vi "Main.vi"(11 "Module Admin":refnum<class "Delacor_lib_QMH_Module Admin.lvclass">) -> ()   [LabVIEW 2024, in "Controller.lvlib"]
doc: "This template is based off of the Queued Message Handler design pattern and the Queued Message Handler project template that ships with LabVIEW.\n\nThe main difference is that the queue is private to this module and communication between modules is performed via Broadcast and Request events.\n\nRequest events are wrapped in public API methods and are handled in the Event Handling Loop (EHL) of this VI. Any module can register for Broadcast events sent by this module. The EHL generates messages based on user interface actions.\n\nThe Message Handling Loop (MHL) processes messages generated by the EHL, or by other messages. The messages are string values, so new messages can be added easily to the Message Cases case structure in the MHL. Each message cluster can also provide an optional value for Message Data, which is a variant that can be converted to whatever message-specific data is required.\n_____\nBased on DQMH Dev Tools: Project Template 7.1.0.1503."
uses:
  Controller.lvlib
  <vilib>/Delacor/Delacor QMH/Libraries/Module Admin_class/Delacor_lib_QMH_Module Admin.lvclass
  Controls/Process state Cluster.ctl
  Controls/Process state enum.ctl
  Module Data--cluster.ctl
  <vilib>/Delacor/Delacor QMH/Libraries/Message Queue_class/Delacor_lib_QMH_Message Queue.lvclass/Delacor_lib_QMH_Message Queue.ctl
  Stop Argument--cluster.ctl
  <vilib>/Delacor/Delacor QMH/Libraries/Module Admin_class/Delacor_lib_QMH_Module Admin.lvclass/Delacor_lib_QMH_Module Admin.ctl
  Login Argument--cluster.ctl
  DB/Controls/Login info.ctl
  DB/Controls/User level.ctl
  Logout Argument--cluster.ctl
  scanner data received Argument--cluster.ctl
  connect all modules Argument--cluster.ctl
  GUI/Controls/Settings.ctl
  <vilib>/Utility/miscctls.llb/LVPointTypeDef.ctl
  <vilib>/Delacor/Delacor QMH/Libraries/Message Queue_class/Delacor_lib_QMH_Enqueue Message (Single).vi
  <vilib>/Delacor/Delacor QMH/Libraries/Module Admin_class/Delacor_lib_QMH_Get External Launch.vi
  <vilib>/Delacor/Delacor QMH/Libraries/Message Queue_class/Delacor_lib_QMH_Message Queue.lvclass
  GUI/GUI.lvlib
  Camera/Camera.lvlib
  DB/DB.lvlib
  Handheld Scanner/Handheld Scanner.lvlib
  PLC/PLC.lvlib
  Aggregation 1/Aggregation 1.lvlib
panel:
  out "scanner read":string
  out "error out":errorcluster
  out "Status":string
  in  "Simulate MHL Error":bool
  in  "Simulate EHL Error":bool
  # "Other processes communicate with this Module via its Public API (wrappers for its Request Events).\n\nThis Module communicates with other processes via its Broadcast Events.\nAny process that wants to receive these messages can register for this module's Broadcast events."
  # "This template is for the DQMH framework. See the block diagram for more information on how to use this template."
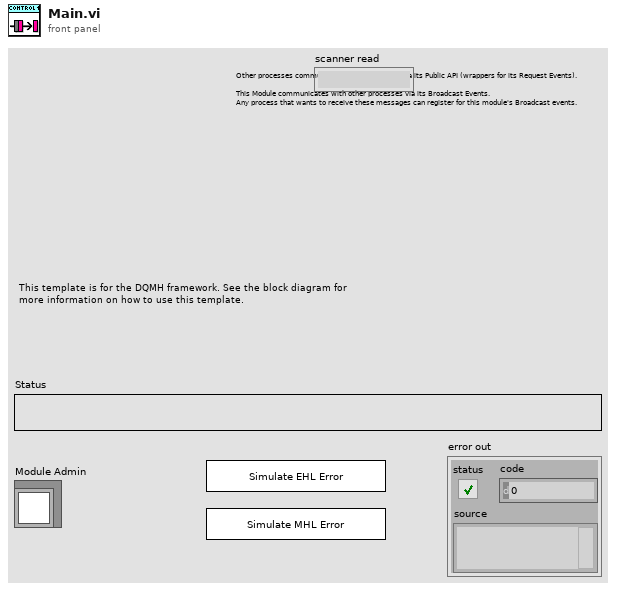
[diagram p1: front panel]
types:
  T1 = typedef "Process state Cluster.ctl" = cluster{T2, variant}
  T2 = typedef "Process state enum.ctl" = enum16{"init", "login", "Agg start", "Agg stop", "logout", "Terminate"}
  T3 = typedef "Controller.lvlib/Request Events--cluster.ctl" = cluster{"Stop Module":refnum<user-event>, "Show Panel":refnum<user-event>, "Hide Panel":refnum<user-event>, "Get Module Execution Status":refnum<user-event>, "Show Diagram":refnum<user-event>, "Login":refnum<user-event>, "Logout":refnum<user-event>, "scanner data received":refnum<user-event>, "connect all modules":refnum<user-event>}
  T4 = typedef "Controller.lvlib/Module Data--cluster.ctl" = cluster{"Status":string}
  T5 = enum32{"invalid lock state", "Not Locked", "Locked (No Password)", "Password-protected"}
  T6 = typedef "Controller.lvlib/Stop Argument--cluster.ctl" = cluster{"Origin":string, "Exit via Stop Module Req?":bool, "Wait for Module to stop?":bool}
  T7 = typedef "Controller.lvlib/Login Argument--cluster.ctl" = cluster{"Login info":T8}
  T8 = typedef "Login info.ctl" = cluster{"User Name":string, "User level":T9}
  T9 = typedef "User level.ctl" = enum16{"Operator", "Admin"}
  T10 = typedef "Controller.lvlib/Logout Argument--cluster.ctl" = cluster{"Boolean":bool}
  T11 = typedef "Controller.lvlib/scanner data received Argument--cluster.ctl" = cluster{"scanner read":string}
  T12 = typedef "Controller.lvlib/connect all modules Argument--cluster.ctl" = cluster{"Settings":T13}
  T13 = typedef "Settings.ctl" = cluster{"Camera 1 IP":string, "Camera 2 IP":string, "Printer 1 IP":string, "Printer 2 IP":string, "Level 2 Scanner COM":refnum<visa-resource-name>, "PLC Port":dbl, "PLC IP":string, "Handheld Scanner COM":refnum<visa-resource-name>, "Printer2 Port":dbl, "Cam1 send port ":dbl, "Cam1 recv port":dbl, "Cam2 send port":dbl, "Cam recv port":dbl, "Printer1 Port":dbl}
  T14 = typedef "LVPointTypeDef.ctl" = cluster{"Horizontal":i16, "Vertical":i16}
  T15 = enum32{"Invalid", "Standard", "Closed", "Hidden", "Minimized", "Maximized"}
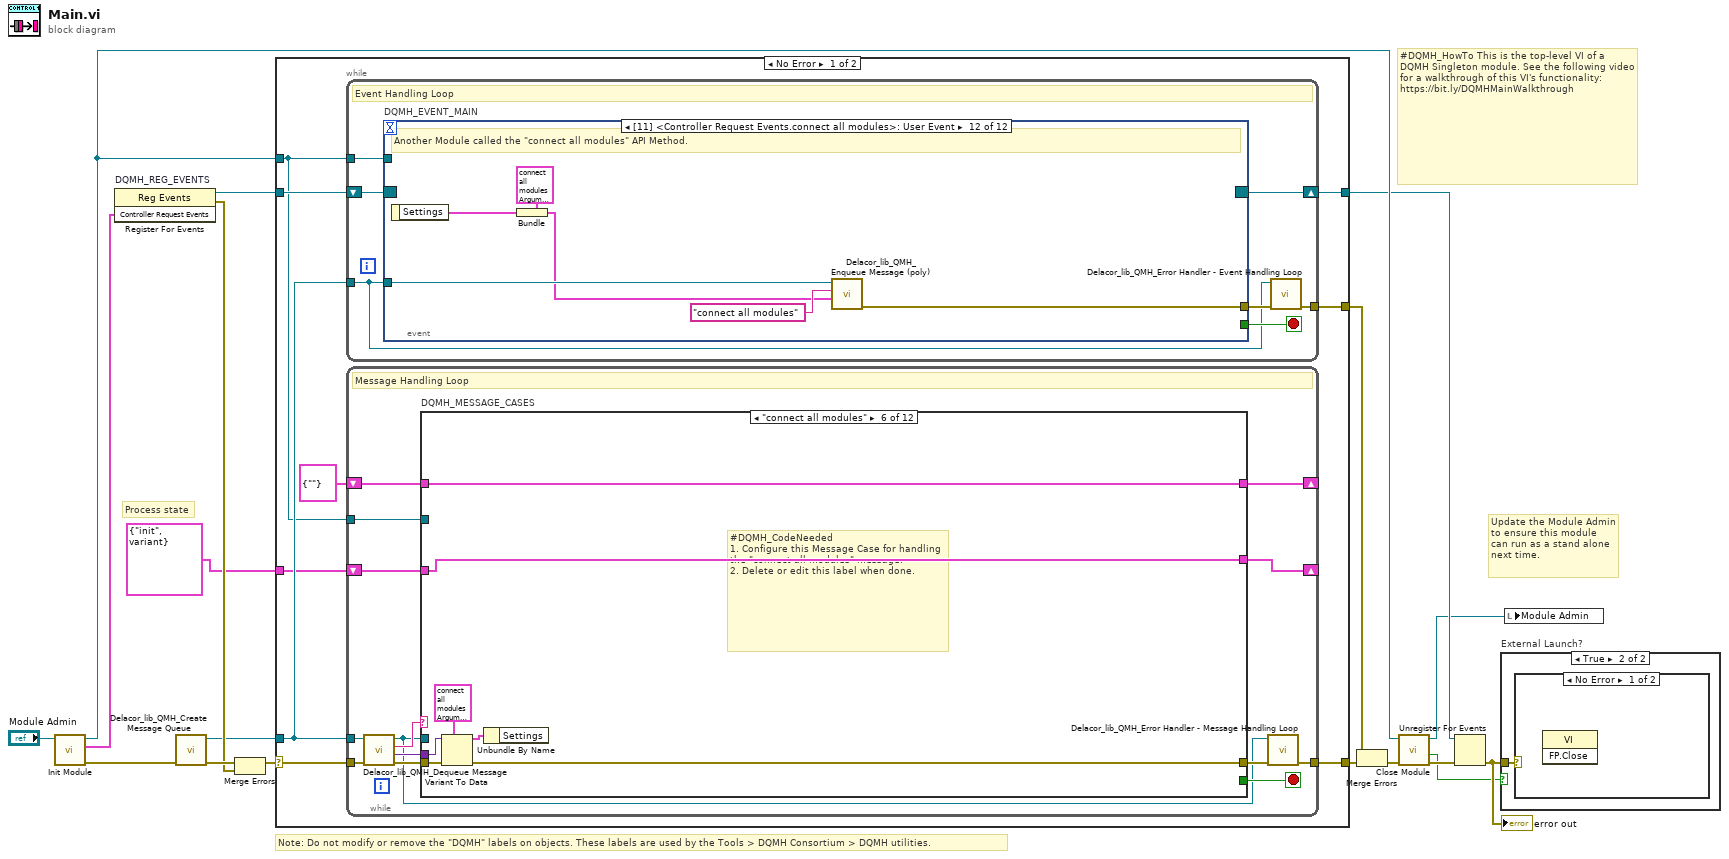
[diagram p0: block diagram]
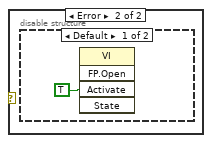
[diagram p3: hidden frame]
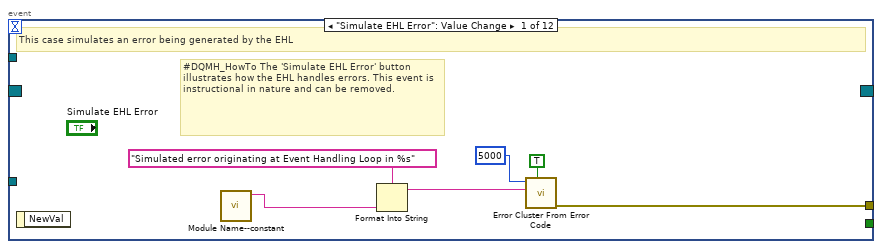
[diagram p5: hidden frame]
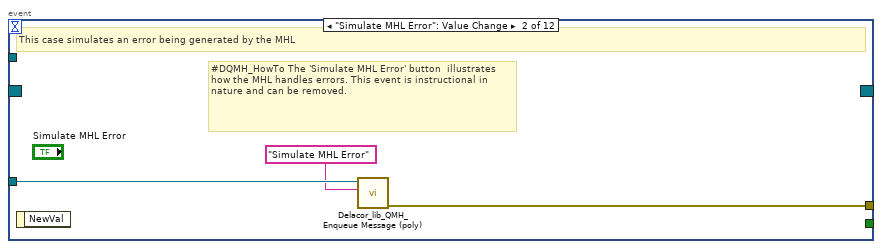
[diagram p6: hidden frame]
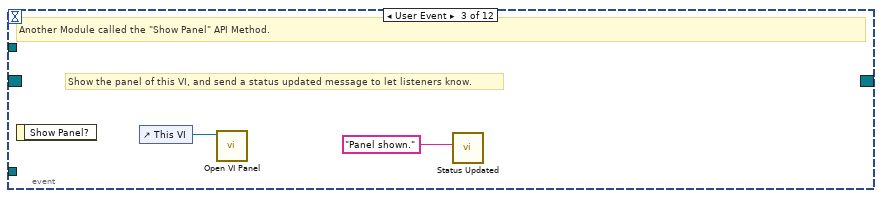
[diagram p7: hidden frame]
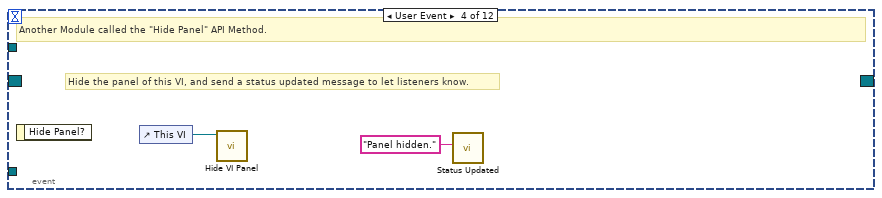
[diagram p8: hidden frame]
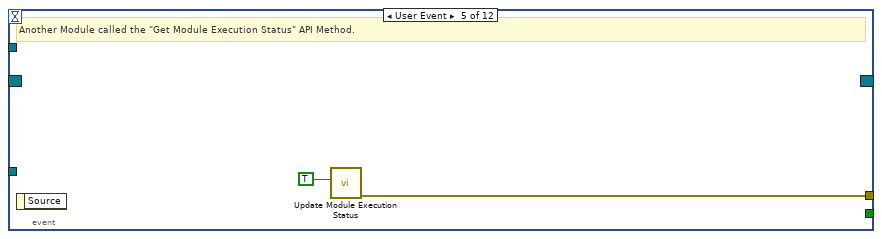
[diagram p9: hidden frame]
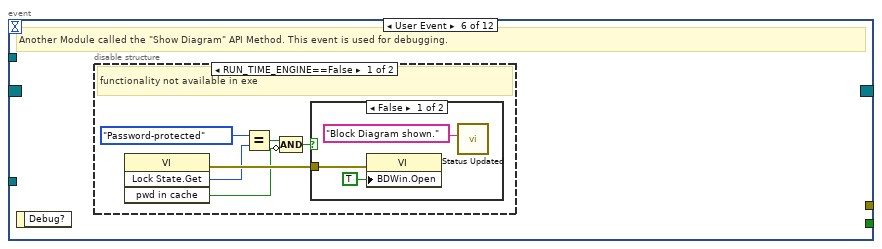
[diagram p10: hidden frame]
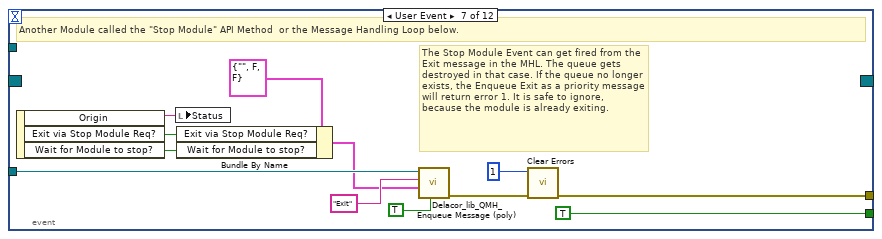
[diagram p13: hidden frame]
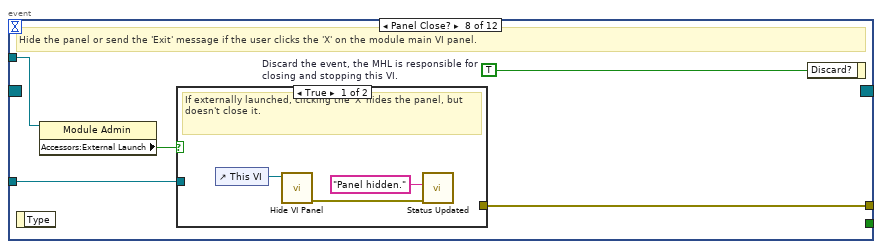
[diagram p14: hidden frame]
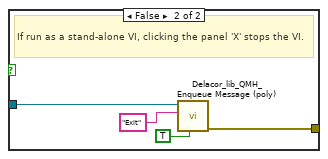
[diagram p15: hidden frame]
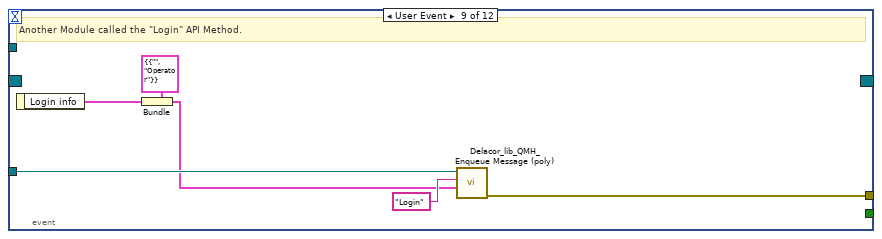
[diagram p16: hidden frame]
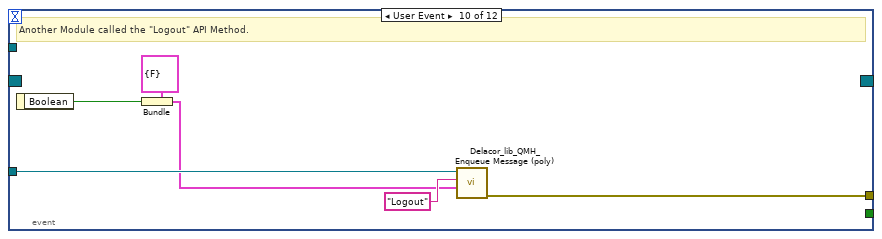
[diagram p17: hidden frame]
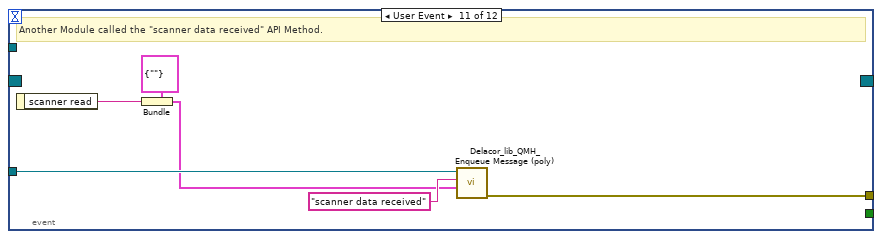
[diagram p18: hidden frame]
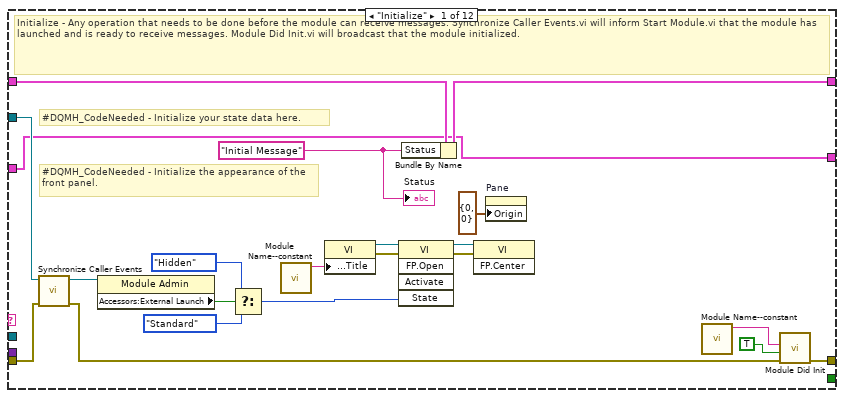
[diagram p19: hidden frame]
diagram:
  # "Process state"
  # "#DQMH_HowTo This is the top-level VI of a DQMH Singleton module. See the following video for a walkthrough of this VI's functionality: https://bit.ly/DQMHMainWalkthrough"
  # "Note: Do not modify or remove the \"DQMH\" labels on objects. These labels are used by the Tools > DQMH Consortium > DQMH utilities."
  # "Update the Module Admin to ensure this module can run as a stand alone next time."
  n1 = call "Init Module.vi"("Singleton Module Admin in"="Module Admin") -> ("error out"=w17:errorcluster, "Controller Request Events"=w6:T3, "Singleton Module Admin out"=w9:refnum<class "Delacor_lib_QMH_Module Admin.lvclass">)  [unwired: 8 in]
  n2 = register-events "DQMH_REG_EVENTS"(w6) -> (reference out=w7:refnum<event-registration>, error out=w10:errorcluster)  [unwired: 2 in]
  n3 = call <vilib>:"Delacor_lib_QMH_Create Message Queue.vi"("error in"=w17) -> ("error out"=w12:errorcluster, "Message Queue"=w5:refnum<class "Delacor_lib_QMH_Message Queue.lvclass">)  [unwired: 9 in]
  n4 = Merge Errors(w12, w10) -> (w11:errorcluster)
  n5 = case shown="No Error" w11 {
    selector: w11 -> [w25 w245]
    tunnel: [w27 w244] -> w18
    tunnel: [w24 w243] -> w8
    tunnel: w7 -> [w22 w243]
    tunnel: w5 -> [w21 w238]
    tunnel: [w26 _] -> w15
    tunnel: w9 -> [w20 w239]
    tunnel: T1 {enum."init", variant} -> [w19 _]
    frame No Error {
      n6 = while {
        tunnel: w21 -> [w28]
        shift-right: [w31] -> w24
        shift-left: w22 -> [w32]
        tunnel: [w33] -> w26
        tunnel: w20 -> [w29]
        stop <- w30 stop-if-true
        # "Event Handling Loop"
        n7 = event "DQMH_EVENT_MAIN" shown="[11] <Controller Request Events.connect all modules>: User Event" {
          selector: w32 -> [_ _ _ _ _ _ _ _ _ _ _ _]
          dyn-events: [_ _ _ _ _ _ _ _ _ _ _ _] -> w31
          timeout: _ -> [_ _ _ _ _ _ _ _ _ _ _ _]
          tunnel: [_ _ _ _ _ _ TRUE ("Discard?") _ _ _ _ _] -> w30
          tunnel: w28 -> [_ w42 _ _ _ _ w66 w73 w88 w94 w100 w106]
          tunnel: [w40 w43 _ _ w49 _ w69 w75 w83 w89 w95 w101] -> w34
          tunnel: w29 -> [_ _ _ _ _ _ _ w72 _ _ _ _]
          event "Simulate EHL Error": Value Change {
            # "#DQMH_HowTo The 'Simulate EHL Error' button  illustrates how the EHL handles errors. This event is instructional in nature and can be removed."
            # "This case simulates an error being generated by the EHL"
            n8 = event-data() -> ()  [unwired: 1 in, 1 out]
            n9 = call "Module Name--constant.vi"() -> ("Module Name"=w37:string)  [unwired: 11 in]
            n10 = Format Into String(format string="Simulated error originating at Event Handling Loop in %s", w37) -> (resulting string=w38:string)  [unwired: 2 in, 1 out]
            n11 = call <vilib>:"Error Cluster From Error Code.vi"("show call chain? (False)"=TRUE, "error message (\"\")"=w38, "error code (0)"=5000) -> ("error out"=w40:errorcluster)  [unwired: 6 in]
          }
          event "Simulate MHL Error": Value Change {
            # "#DQMH_HowTo The 'Simulate MHL Error' button  illustrates how the MHL handles errors. This event is instructional in nature and can be removed."
            # "This case simulates an error being generated by the MHL"
            n12 = event-data() -> ()  [unwired: 1 in, 1 out]
            n13 = call-poly <vilib>:"Delacor_lib_QMH_Enqueue Message (poly).vi"("Message"="Simulate MHL Error", "Message Queue in"=w42) -> ("error out"=w43:errorcluster)  [unwired: 8 in, 1 out]
          }
          event User Event {
            # "Show the panel of this VI, and send a status updated message to let listeners know."
            # "Another Module called the \"Show Panel\" API Method."
            n14 = event-data() -> ()  [unwired: 1 in, 1 out]
            n15 = control-ref of="This VI"() -> (w45:refnum<vi>)
            n16 = call "Open VI Panel.vi"("VI"=w45) -> ()  [unwired: 10 in, 1 out]
            n17 = call "Status Updated.vi"("Status"="Panel shown." ("format string")) -> ()  [unwired: 10 in, 1 out]
          }
          event User Event {
            # "Hide the panel of this VI, and send a status updated message to let listeners know."
            # "Another Module called the \"Hide Panel\" API Method."
            n18 = event-data() -> ()  [unwired: 1 in, 1 out]
            n19 = control-ref of="This VI"() -> (w47:refnum<vi>)
            n20 = call "Hide VI Panel.vi"("VI"=w47) -> ()  [unwired: 10 in, 1 out]
            n21 = call "Status Updated.vi"("Status"="Panel hidden." ("format string")) -> ()  [unwired: 10 in, 1 out]
          }
          event User Event {
            # "Another Module called the \"Get Module Execution Status\" API Method."
            n22 = event-data() -> ()  [unwired: 1 in, 1 out]
            n23 = call "Update Module Execution Status.vi"("Running?"=TRUE) -> ("error out"=w49:errorcluster)  [unwired: 10 in]
          }
          event User Event {
            # "Another Module called the \"Show Diagram\" API Method. This event is used for debugging."
            n24 = event-data() -> ()  [unwired: 1 in, 1 out]
            n25 = disable-structure shown="RUN_TIME_ENGINE==False" {
              frame condition #0 (active) {
                # "functionality not available in exe"
                n26 = invoke on="Invoke Node" class="VI" method="Lock State.Get"() -> (error out=w55:errorcluster, "Get Lock State"=w54:T5, "pwd in cache"=w51:bool)  [unwired: 4 in, 1 out]
                n27 = Equal?(x=T5."Password-protected", y=w54) -> (x = y?=w52:bool)
                n28 = Compound Arithmetic op=AND(w52, invert w51) -> (w50:bool)
                n29 = case shown="False" w50 {
                  tunnel: w55 -> [w58 _]
                  frame False {
                    n30 = property on="Property Node" class="VI"(error in=w58, "BDWin.Open"=TRUE ("Block Diagram Window:Open")) -> ()  [unwired: 1 in, 2 out]
                    n31 = call "Status Updated.vi"("Status"="Block Diagram shown." ("format string")) -> ()  [unwired: 10 in, 1 out]
                  }
                  frame True {
                    # "Password-protected VI, and the password is not in the cache. Do not show the diagram."
                  }
                }
              }
              frame condition #1 {
              }
            }
          }
          event User Event {
            # "The Stop Module Event can get fired from the Exit message in the MHL. The queue gets destroyed in that case. If the queue no longer exists, the Enqueue Exit as a priority message will return error 1. It is safe to ignore, because the module is already exiting."
            # "Another Module called the \"Stop Module\" API Method  or the Message Handling Loop below."
            n32 = event-data() -> ("Origin"=w65:string, "Exit via Stop Module Req?"=w61:bool, "Wait for Module to stop?"=w60:bool)  [unwired: 1 in]
            n33 = local write "Status"(w65) -> ()
            n34 = Bundle By Name(cluster=T6 {"Origin"="", "Exit via Stop Module Req?"=FALSE, "Wait for Module to stop?"=FALSE} ("Stop Argument"), "Exit via Stop Module Req?"=w61, "Wait for Module to stop?"=w60) -> (w59:T6)
            n35 = call-poly <vilib>:"Delacor_lib_QMH_Enqueue Message (poly).vi"("Priority Message? (F)"=TRUE, "Message Data"=w59, "Message"="Exit", "Message Queue in"=w66) -> ("error out"=w70:errorcluster)  [unwired: 6 in, 1 out]
            n36 = call <vilib>:"Clear Errors.vi"("error in (no error)"=w70, "specific error code to clear (0: all)"=1) -> ("error out"=w69:errorcluster)  [unwired: 4 in, 1 out]
          }
          event Panel Close? {
            w74 = TRUE  # Discard the event, the MHL is responsible for closing and stopping this VI.
            # "Hide the panel or send the 'Exit' message if the user clicks the 'X' on the module main VI panel."
            n37 = event-data() -> ()  [unwired: 1 in, 1 out]
            n38 = property on="Property Node" class="Module Admin"(reference=w72) -> ("Accessors:External Launch"=w71:bool)  [unwired: 1 in, 2 out]
            n39 = case shown="True" w71 {
              tunnel: w73 -> [_ w81]
              tunnel: [_ w82] -> w75
              frame True {
                # "If externally launched, clicking the 'X' hides the panel, but doesn't close it."
                n40 = control-ref of="This VI"() -> (w78:refnum<vi>)
                n41 = call "Hide VI Panel.vi"("VI"=w78) -> ("error out"=w76:errorcluster)  [unwired: 10 in]
                n42 = call "Status Updated.vi"("error in"=w76, "Status"="Panel hidden." ("format string")) -> ()  [unwired: 9 in, 1 out]
              }
              frame False {
                # "If run as a stand-alone VI, clicking the panel 'X' stops the VI."
                n43 = call-poly <vilib>:"Delacor_lib_QMH_Enqueue Message (poly).vi"("Priority Message? (F)"=TRUE, "Message"="Exit", "Message Queue in"=w81) -> ("error out"=w82:errorcluster)  [unwired: 7 in, 1 out]
              }
            }
            n44 = event-data ("Event Filter Node")("Discard?"=w74) -> ()  [unwired: 1 in, 1 out]
          }
          event User Event {
            # "Another Module called the \"Login\" API Method."
            n45 = event-data() -> ("Login info"=w84:T8)  [unwired: 1 in]
            n46 = Bundle(cluster=T7 {"Login info"={"User Name"="", "User level"=enum."Operator"}} ("Login Argument"), "Login info"=w84) -> (w85:T7)
            n47 = call-poly <vilib>:"Delacor_lib_QMH_Enqueue Message (poly).vi"("Message Data"=w85, "Message"="Login", "Message Queue in"=w88) -> ("error out"=w83:errorcluster)  [unwired: 7 in, 1 out]
          }
          event User Event {
            # "Another Module called the \"Logout\" API Method."
            n48 = event-data() -> ("Boolean"=w90:bool)  [unwired: 1 in]
            n49 = Bundle(cluster=T10 {"Boolean"=FALSE} ("Logout Argument"), "Boolean"=w90) -> (w91:T10)
            n50 = call-poly <vilib>:"Delacor_lib_QMH_Enqueue Message (poly).vi"("Message Data"=w91, "Message"="Logout", "Message Queue in"=w94) -> ("error out"=w89:errorcluster)  [unwired: 7 in, 1 out]
          }
          event User Event {
            # "Another Module called the \"scanner data received\" API Method."
            n51 = event-data() -> ("scanner read"=w96:string)  [unwired: 1 in]
            n52 = Bundle(cluster=T11 {"scanner read"=""} ("scanner data received Argument"), "scanner read"=w96) -> (w97:T11)
            n53 = call-poly <vilib>:"Delacor_lib_QMH_Enqueue Message (poly).vi"("Message Data"=w97, "Message"="scanner data received", "Message Queue in"=w100) -> ("error out"=w95:errorcluster)  [unwired: 7 in, 1 out]
          }
          event User Event {
            # "Another Module called the \"connect all modules\" API Method."
            n54 = event-data() -> ("Settings"=w102:T13)  [unwired: 1 in]
            n55 = Bundle(cluster=T12 {"Settings"={"Camera 1 IP"="", "Camera 2 IP"="", "Printer 1 IP"="", "Printer 2 IP"="", "Level 2 Scanner COM"="", "PLC Port"=0.0, "PLC IP"="", "Handheld Scanner COM"="", "Printer2 Port"=0.0, "Cam1 send port "=0.0, "Cam1 recv port"=0.0, "Cam2 send port"=0.0, "Cam recv port"=0.0, "Printer1 Port"=0.0}} ("connect all modules Argument"), "Settings"=w102) -> (w103:T12)
            n56 = call-poly <vilib>:"Delacor_lib_QMH_Enqueue Message (poly).vi"("Message Data"=w103, "Message"="connect all modules", "Message Queue in"=w106) -> ("error out"=w101:errorcluster)  [unwired: 7 in, 1 out]
          }
        }
        n57 = call-dynamic "Delacor_lib_QMH_Error Handler - Event Handling Loop.vi"("error in"=w34, "Message Queue in"=w28) -> ("dup error in"=w33:errorcluster)  [unwired: 8 in, 1 out]
      }
      n58 = while {
        tunnel: w21 -> [w109]
        shift-right: [w117] -> _
        shift-left: T4 {"Status"=""} ("Data Cluster") -> [w118]
        tunnel: w25 -> [w120]
        tunnel: [w112] -> w27
        tunnel: w20 -> [w113]
        shift-right: [w107] -> _
        shift-left: w19 -> [w108]
        stop <- w116 stop-if-true
        # "Message Handling Loop"
        n59 = call-dynamic "Delacor_lib_QMH_Dequeue Message.vi"("error in"=w120, "Message Queue in"=w109) -> ("error out"=w119:errorcluster, "Message Data"=w114:variant, "Message"=w115:string, "Message Queue out"=w110:refnum<class "Delacor_lib_QMH_Message Queue.lvclass">)  [unwired: 6 in]
        n60 = case "DQMH_MESSAGE_CASES" shown="\"connect all modules\"" w115 {
          selector: w115 -> [_ _ _ _ _ _ _ _ _ _ _ w233]
          tunnel: w110 -> [_ _ _ _ _ _ _ _ _ w196 w220 _]
          tunnel: w119 -> [w139 w144 w152 w159 w167 w174 w178 w181 w191 w203 w226 w236]
          tunnel: [w137 w144 w150 w157 w165 w171 w177 w181 w190 w199 w221 w237] -> w111
          tunnel: w118 -> [w128 w143 w151 w158 w166 w173 w176 w180 w188 w198 w219 w234]
          tunnel: [w127 w143 w151 w158 w166 w173 w176 w180 w188 w198 w219 w234] -> w117
          tunnel: [_ _ _ _ _ _ _ _ _ _ w218 _] -> w116
          tunnel: w114 -> [_ _ w149 w156 w164 w170 _ _ _ w197 w217 _]
          tunnel: w113 -> [w129 _ _ _ _ _ _ _ _ w195 w212 _]
          tunnel: w108 -> [w121 w142 _ w153 w160 w172 w175 w179 w182 w192 w210 w227]
          tunnel: [w121 w142 T1 {enum."login", variant} w153 w160 w172 w175 w179 w182 w192 w210 w227] -> w107
          frame "Initialize" {
            w123 = "Initial Message" ("Initial Message")
            # "#DQMH_CodeNeeded - Initialize the appearance of the front panel."
            # "#DQMH_CodeNeeded - Initialize your state data here."
            # "Initialize - Any operation that needs to be done before the module can receive messages. Synchronize Caller Events.vi will inform Start Module.vi that the module has launched and is ready to receive messages. Module Did Init.vi will broadcast that the module initialized."
            n61 = call "Synchronize Caller Events.vi"("error in"=w139, "Singleton Module Admin in"=w129) -> ("error out"=w138:errorcluster, "Singleton Module Admin out"=w124:refnum<class "Delacor_lib_QMH_Module Admin.lvclass">)  [unwired: 8 in]
            n62 = property on="Property Node" class="Module Admin"(reference=w124) -> ("Accessors:External Launch"=w133:bool)  [unwired: 1 in, 2 out]
            n63 = Select(t=T15."Hidden" ("State"), s=w133, f=T15."Standard" ("State")) -> (s? t:f=w130:T15)
            n64 = call "Module Name--constant.vi"() -> ("Module Name"=w136:string)  [unwired: 11 in]
            n65 = property on="Property Node" class="VI"("Front Panel.Title"=w136) -> (reference out=w135:refnum<vi>, error out=w141:errorcluster)  [unwired: 2 in]
            n66 = invoke on="Invoke Node" class="VI" method="FP.Open"(reference=w135, error in=w141, "State"=w130) -> (reference out=w134:refnum<vi>, error out=w140:errorcluster)  [unwired: 2 in, 3 out]
            n67 = Bundle By Name(cluster=w128, "Status"=w123) -> (w127:T4)
            n68 = invoke on="Invoke Node" class="VI" method="FP.Center"(reference=w134, error in=w140) -> ()  [unwired: 1 in, 3 out]
            n69 = property on="Pane" class="Pane"("Origin"=T14 {"Horizontal"=0, "Vertical"=0}) -> ()  [unwired: 2 in, 2 out]
            n70 = call "Module Name--constant.vi"() -> ("Module Name"=w125:string)  [unwired: 11 in]
            n71 = call "Module Did Init.vi"("error in"=w138, "Initialized?"=TRUE, "Origin"=w125) -> ("error out"=w137:errorcluster)  [unwired: 8 in]
            "Status" <- w123
          }
          frame "---Module Specific---" {
            # "Separator -- The following cases handle messages specific to this Module."
          }
          frame "Login" {
            n72 = Variant To Data(error in=w152, type=T7 {"Login info"={"User Name"="", "User level"=enum."Operator"}} ("Login Argument"), Variant=w149) -> (data=w147:T7, error out=w150:errorcluster)
            n73 = Unbundle By Name(w147) -> ("Login info"=w146:T8)
            n74 = call "login_.vi"("Login info"=w146) -> ()  [unwired: 10 in, 1 out]
          }
          frame "Logout" {
            n75 = Variant To Data(error in=w159, type=T10 {"Boolean"=FALSE} ("Logout Argument"), Variant=w156) -> (data=w154:T10, error out=w157:errorcluster)
            n76 = Unbundle By Name(w154) -> ()  [unwired: 1 out]
            n77 = call "logout.vi"() -> ()  [unwired: 11 in, 1 out]
          }
          frame "scanner data received" {
            # "#DQMH_CodeNeeded\n1. Configure this Message Case for handling the \"scanner data received\" message.\n2. Delete or edit this label when done."
            n78 = Variant To Data(error in=w167, type=T11 {"scanner read"=""} ("scanner data received Argument"), Variant=w164) -> (data=w162:T11, error out=w165:errorcluster)
            n79 = Unbundle By Name(w162) -> ("scanner read"=→"scanner read":string)
          }
          frame "connect all modules" {
            # "#DQMH_CodeNeeded\n1. Configure this Message Case for handling the \"connect all modules\" message.\n2. Delete or edit this label when done."
            n80 = Variant To Data(error in=w174, type=T12 {"Settings"={"Camera 1 IP"="", "Camera 2 IP"="", "Printer 1 IP"="", "Printer 2 IP"="", "Level 2 Scanner COM"="", "PLC Port"=0.0, "PLC IP"="", "Handheld Scanner COM"="", "Printer2 Port"=0.0, "Cam1 send port "=0.0, "Cam1 recv port"=0.0, "Cam2 send port"=0.0, "Cam recv port"=0.0, "Printer1 Port"=0.0}} ("connect all modules Argument"), Variant=w170) -> (data=w168:T12, error out=w171:errorcluster)
            n81 = Unbundle By Name(w168) -> ()  [unwired: 1 out]
          }
          frame "---Copy This Frame---" {
            # "Duplicate this frame when creating new messages.  Change this comment in the duplicated frame to describe this message."
            n82 = Merge Errors(w178) -> (w177:errorcluster)
          }
          frame "---Exit and Error Handling---" {
            # "Separator - The following cases handle errors and exit messages."
          }
          frame "Simulate MHL Error" {
            # "#DQMH_HowTo The 'Simulate MHL Error' button  illustrates how the MHL handles errors. This event is instructional in nature and can be removed."
            # "Simulate an error occurring at the MHL"
            n83 = call "Module Name--constant.vi"() -> ("Module Name"=w184:string)  [unwired: 11 in]
            n84 = Format Into String(format string="Simulated error originating at Message Handling Loop in %s", w184) -> (resulting string=w185:string)  [unwired: 2 in, 1 out]
            n85 = call <vilib>:"Error Cluster From Error Code.vi"("show call chain? (False)"=TRUE, "error message (\"\")"=w185, "error code (0)"=5001) -> ("error out"=w189:errorcluster)  [unwired: 6 in]
            n86 = Merge Errors(w191, w189) -> (w190:errorcluster)
          }
          frame "Error" {
            # "#DQMH_CodeRecommended - If the module is running in standalone mode (External Launch = FALSE), this code will pop up an error dialog and call the 'Exit' message if an error occurs. Add more fine-grained error management here."
            # "Error - Check the error message data and respond accordingly. This message is sent by the \"Error Handler\" VIs at the end of each loop in this application."
            n87 = property on="Property Node" class="Module Admin"(reference=w195) -> ("Accessors:External Launch"=w194:bool)  [unwired: 1 in, 2 out]
            n88 = Variant To Data(error in=w203, type=errorcluster {"status"=FALSE, "code"=0, "source"=""} ("error constant"), Variant=w197) -> (data=w193:errorcluster, error out=w201:errorcluster)
            n89 = local write "error out"(w193) -> ()
            n90 = call "Error Reported.vi"("Error"=w193) -> ()  [unwired: 10 in, 1 out]
            n91 = case shown="False" w194 {
              tunnel: [w208 _] -> w200
              tunnel: w196 -> [w206 _]
              tunnel: w193 -> [w207 _]
              frame False {
                n92 = disable-structure shown="Default" {
                  disable-tunnel: w207 -> [w209 _]
                  frame condition #0 (active) {
                    # "If the module is running standalone, then pop up an error dialog and call the \"Exit\" message."
                    n93 = call <vilib>:"Simple Error Handler.vi"("error in (no error)"=w209) -> ()  [unwired: 4 in, 5 out]
                  }
                  frame condition #1 {
                    # "To prevent the Simple Error Handler VI from being loaded (e.g. when deploying to a Real-Time target), add the Conditional Disable Symbol \"DQMH_Disable_SEH\" to your project and set it to TRUE."
                  }
                }
                n94 = call-poly <vilib>:"Delacor_lib_QMH_Enqueue Message (poly).vi"("Priority Message? (F)"=TRUE, "Message"="Exit", "Message Queue in"=w206) -> ("error out"=w208:errorcluster)  [unwired: 7 in, 1 out]
              }
              frame True {
                # "If the module was launched externally, calling the Error Reported broadcast VI is the only action performed by the \"Error\" message. The module's caller can then process the error appropriately."
              }
            }
            n95 = Merge Errors(w201, w200) -> (w199:errorcluster)
          }
          frame "Exit" {
            w216 = 91  # 91: not all Exit messages will have an argument
            w218 = TRUE  # Stop the VI
            # "Closing all modules"
            # "Release the message queue reference"
            # "#DQMH_CodeNeeded - Add any required cleanup code here."
            # "Exit - Exit the application."
            n96 = Variant To Data(error in=w226, type=T6 {"Origin"="", "Exit via Stop Module Req?"=FALSE, "Wait for Module to stop?"=FALSE} ("Stop Argument"), Variant=w217) -> (data=w214:T6, error out=w223:errorcluster)
            n97 = call <vilib>:"Clear Errors.vi"("error in (no error)"=w223, "specific error code to clear (0: all)"=w216) -> ("error out"=w225:errorcluster)  [unwired: 4 in, 1 out]
            n98 = control-ref of="This VI"() -> (w213:refnum<vi>)
            n99 = call-dynamic "Delacor_lib_QMH_Release Message Queue.vi"("error in"=w225, "Message Queue"=w220) -> ("error out"=w224:errorcluster)  [unwired: 9 in]
            n100 = call "Handle Exit.vi"("Stop Argument"=w214, "Admin in"=w212, "VI reference"=w213) -> ("error out"=w222:errorcluster)  [unwired: 7 in, 1 out]
            n101 = Merge Errors(w224, w222) -> (w221:errorcluster)
            n102 = call "Error Reported.vi"("Error"=w221) -> ()  [unwired: 10 in, 1 out]
            n103 = call "Stop Module.vi"("Module ID"=-1) -> ()  [unwired: 10 in, 1 out]
            n104 = call "Stop Module.vi"() -> ()  [unwired: 11 in, 1 out]
            n105 = call "Stop Module.vi"() -> ()  [unwired: 11 in, 1 out]
            n106 = call "Stop Module.vi"() -> ()  [unwired: 11 in, 1 out]
            n107 = call "Stop Module.vi"() -> ()  [unwired: 11 in, 1 out]
          }
          frame Default {
            # "'Default' case only runs if there is a message that isn't defined in any of the other cases.  Output a programming error."
            n108 = call "Module Name--constant.vi"() -> ("Module Name"=w232:string)  [unwired: 11 in]
            n109 = Format Into String(format string="The invalid message string \"%s\" was received in the Message Handling Loop for module \"%s\".", w233, w232) -> (resulting string=w228:string)  [unwired: 2 in, 1 out]
            n110 = call <vilib>:"Error Cluster From Error Code.vi"("show call chain? (False)"=TRUE, "error message (\"\")"=w228, "error code (0)"=1) -> ("error out"=w235:errorcluster)  [unwired: 6 in]
            n111 = Merge Errors(w236, w235) -> (w237:errorcluster)
          }
        }
        n112 = call-dynamic "Delacor_lib_QMH_Error Handler - Message Handling Loop.vi"("error in"=w111, "Message Queue in"=w110) -> ("dup error in"=w112:errorcluster)  [unwired: 8 in, 1 out]
      }
    }
    frame Error {
      # "Synchronize Caller Events.vi will inform Start Module.vi that the module has launched and will let the code calling Start Module.vi register for broadcasts and would permit the caller receive the broadcast that an error occurred at launch time."
      n113 = call-dynamic "Delacor_lib_QMH_Release Message Queue.vi"("error in"=w245, "Message Queue"=w238) -> ("error out"=w244:errorcluster)  [unwired: 9 in]
      n114 = call "Synchronize Caller Events.vi"("Singleton Module Admin in"=w239) -> ("error out"=w246:errorcluster)  [unwired: 9 in, 1 out]
      n115 = call "Module Name--constant.vi"() -> ("Module Name"=w242:string)  [unwired: 11 in]
      n116 = Format Into String(format string="An error occurred during initialization. %s is no longer running.", w242) -> (resulting string=w240:string)  [unwired: 2 in, 1 out]
      n117 = Merge Errors(w244, w246) -> (w247:errorcluster)
      n118 = call "Error Reported.vi"("Additional Information"=w240, "Error"=w247) -> ()  [unwired: 9 in, 1 out]
    }
  }
  n119 = Merge Errors(w15, w18) -> (w14:errorcluster)
  n120 = call "Close Module.vi"("error in"=w14, "Module Admin in"=w9) -> ("error out"=w16:errorcluster, "External Launch"=w2:bool, "Module Admin out"=w3:refnum<class "Delacor_lib_QMH_Module Admin.lvclass">)  [unwired: 7 in]
  n121 = Unregister For Events(event registration refnum=w8, error in=w16) -> (error out=w13:errorcluster)
  "error out" <- w13
  n122 = case "External Launch?" shown="True" w2 {
    tunnel: w13 -> [_ w248]
    frame False {
    }
    frame True {
      n123 = case shown="No Error" w248 {
        frame No Error {
          n124 = invoke on="Invoke Node" class="VI" method="FP.Close"() -> ()  [unwired: 3 in, 3 out]
        }
        frame Error {
          n125 = disable-structure shown="Default" {
            frame condition #0 (active) {
              n126 = invoke class="VI" method="FP.Open"("Activate"=TRUE ("Activate?")) -> ()  [unwired: 4 in, 5 out]
            }
            frame condition #1 {
              # "Don't show panel on error if running inside a built EXE."
            }
          }
        }
      }
    }
  }
  n127 = local write "Module Admin"(w3) -> ()
